vi "Gen - Poup Key in Sequence.vi"(6 "Type":enum16{"Error", "Info"}(ring)=enum."Info", 8 "Error in":errorcluster, 9 "Button text":string[](array[string])=["YES", "NO"], 10 "Data in":string[](array[string])) -> (0 "Error out":errorcluster, 2 "Data Out":T1, 3 "Yes?":bool)   [LabVIEW 2020]
uses:
  Control/State - eFGV.ctl
panel:
  in  "Section":string
  in  "Max blowdown pressure (psi)":string
  in  "Actuator pressure (psi)":string
  in  "Blowdown (Y/N)":string
  in  "Chart scale":string
  in  "Holding Time":string
  in  "Cycle":string(combo)
  in  "Test Pressure (psi)":string
  in  "Test Bunker":string(combo)
  in  "Test Media":string
  in  "Test Procedure":string
  in  "Variance":string
  in  "Test Req.":string
  in  "Test Req. ID":string
  in  "Test Sequence":string
  in  "Current File name":string
  out "procedure no./ref.  filename":string
  in  "Template Name":string
  out "Type Error":bool
  in  "No":bool
  in  "Yes":bool
  in  "Cancel":bool
  out "Type Info":bool
  in  "OK":bool
  out "Header out":string
  in  "Exit":bool
  out "Message":string
  in  "Auto Close?":bool
  in  "Message in":string
  in  "Header":string
  # "Sequence Parameter"
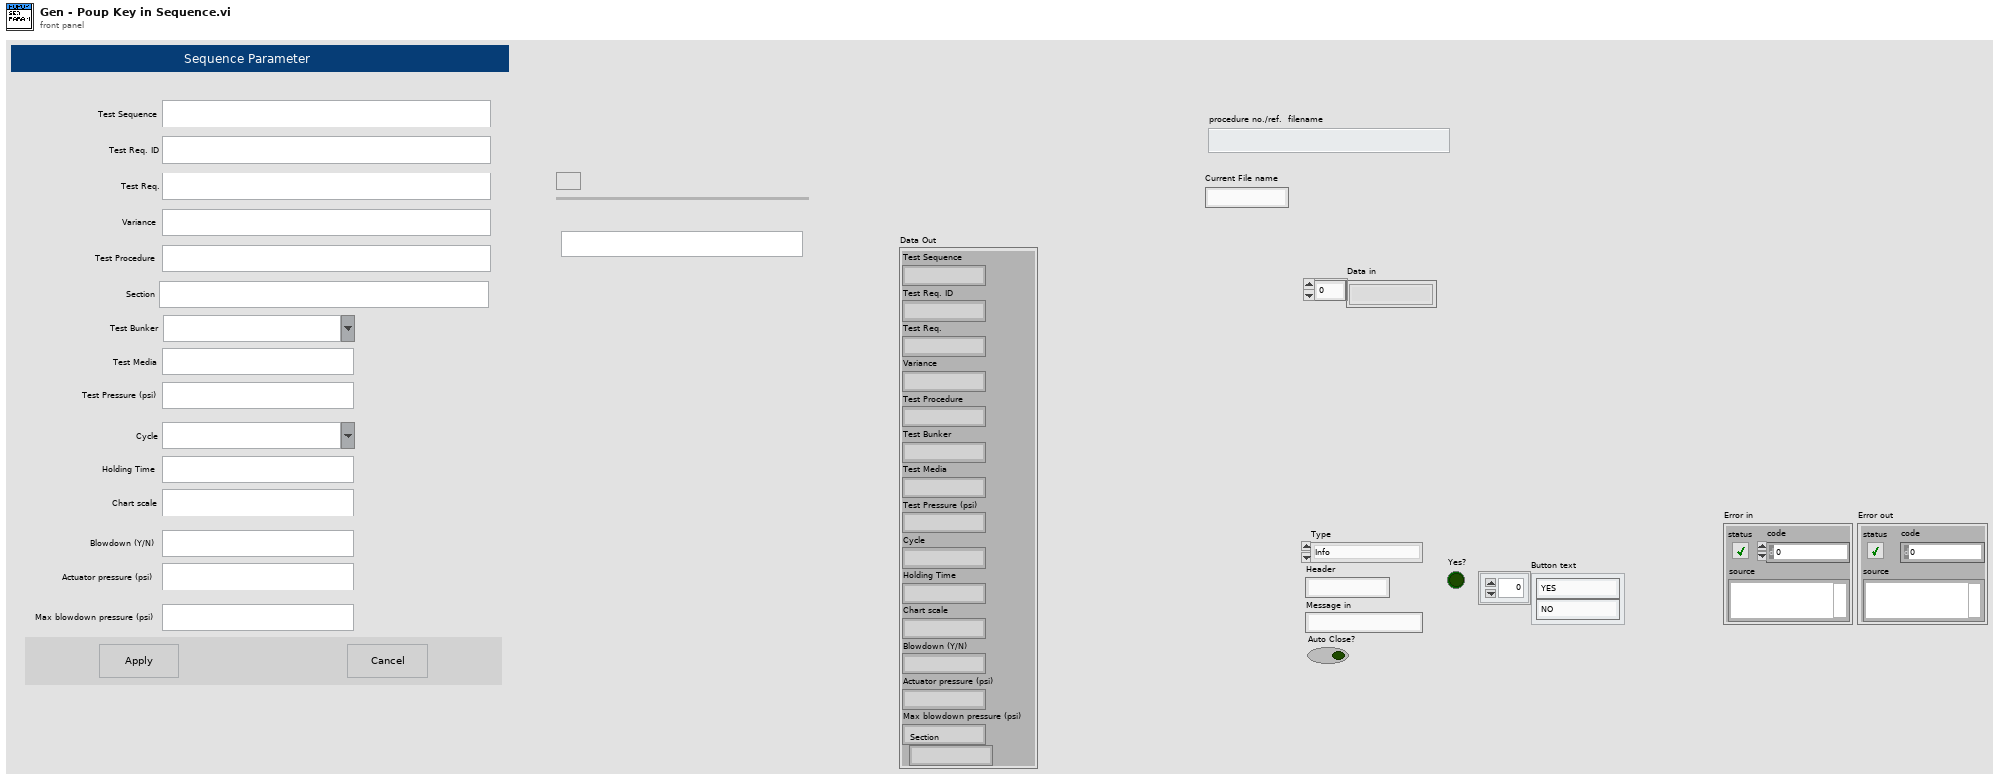
[diagram p1: front panel]
types:
  T1 = cluster{"Test Sequence":string, "Test Req. ID":string, "Test Req.":string, "Variance":string, "Test Procedure":string, "Test Bunker":string, "Test Media":string, "Test Pressure (psi)":string, "Cycle":string, "Holding Time":string, "Chart scale":string, "Blowdown (Y/N)":string, "Actuator pressure (psi)":string, "Max blowdown pressure (psi)":string, "Section":string}
  T2 = typedef "State - eFGV.ctl" = enum16{"Init", "Read", "Write", "Exit"}
  T3 = enum32{"Invalid", "Default", "Floating", "Floating/Auto-Hide", "Modal"}
  T4 = enum8{"Enabled", "Disabled", "Disabled and Grayed Out"}
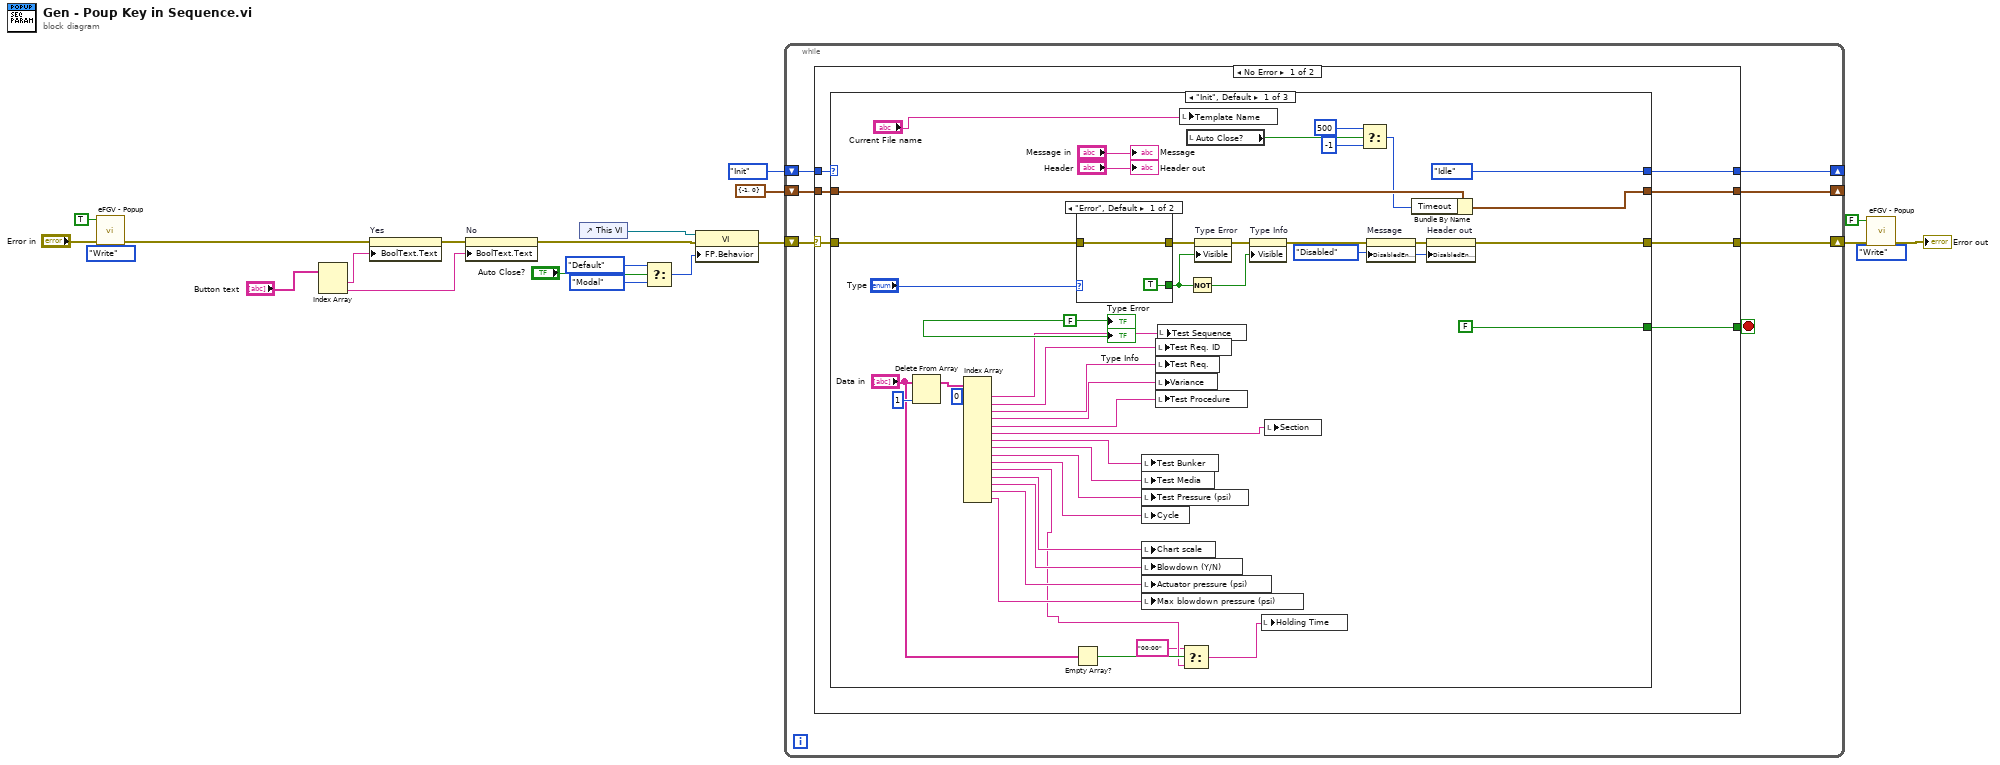
[diagram p0: block diagram]
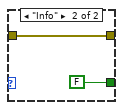
[diagram p2: hidden frame]
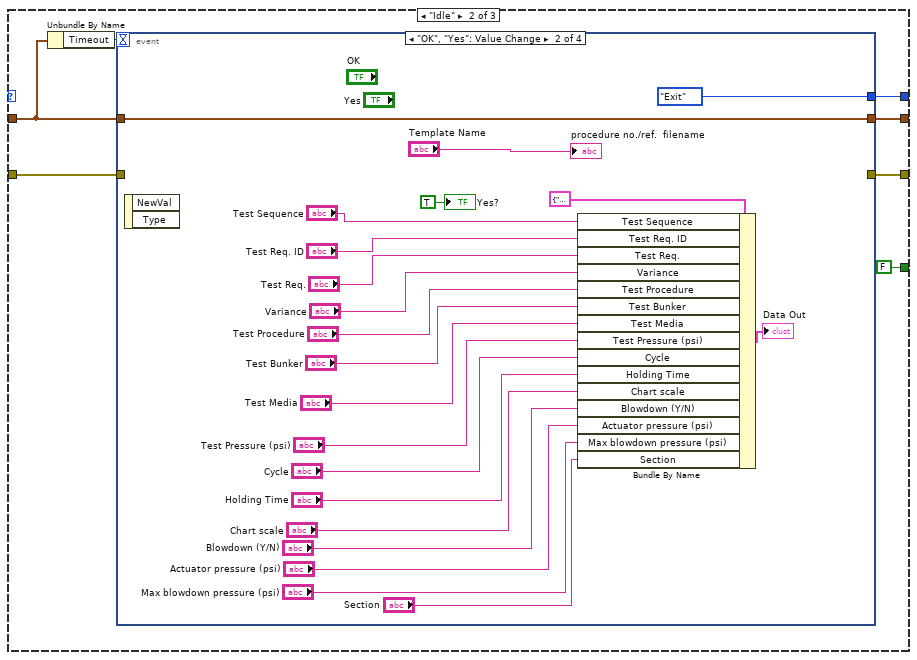
[diagram p3: hidden frame]
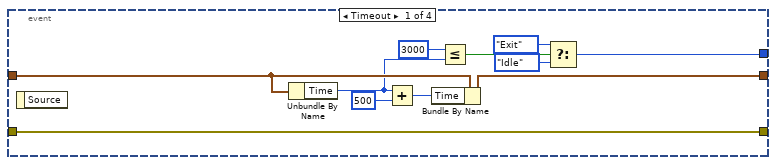
[diagram p4: hidden frame]
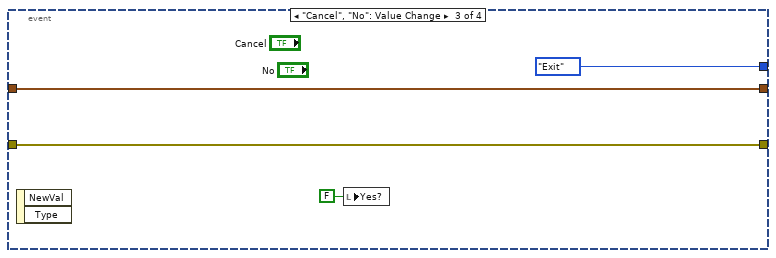
[diagram p5: hidden frame]
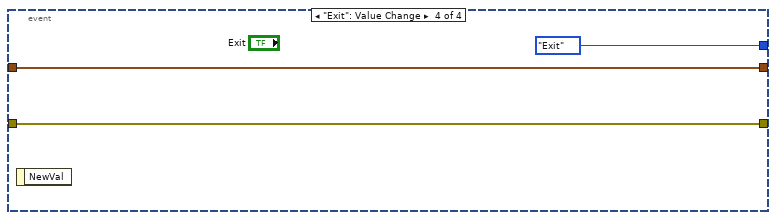
[diagram p6: hidden frame]
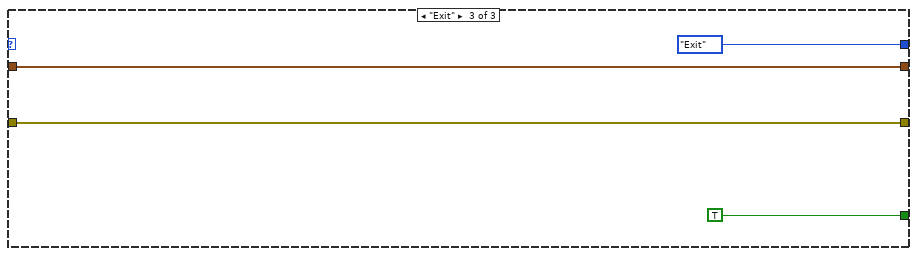
[diagram p7: hidden frame]
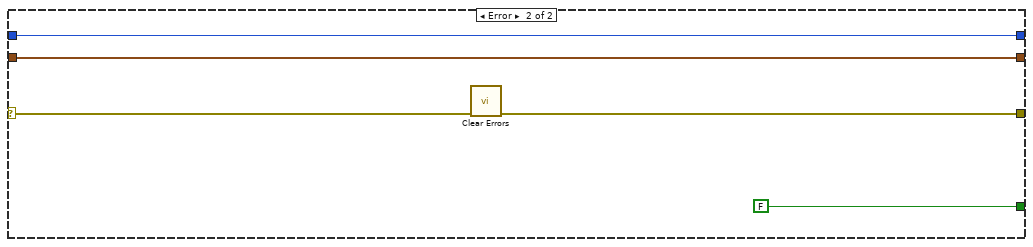
[diagram p8: hidden frame]
diagram:
  n1 = call "eFGV - Popup.vi"("Action"=State_-_eFGV."Write", "Error In"="Error in", "Popup"=TRUE) -> ("Error Out"=w1:errorcluster)  [unwired: 6 in, 2 out]
  n2 = Index Array(array="Button text") -> (element #1=w10:string, element #2=w9:string)  [unwired: 2 in]
  n3 = property on="Yes" class="Bool"(error in=w1, "BoolText.Text"=w10) -> (error out=w13:errorcluster)  [unwired: 1 in, 1 out]
  n4 = property on="No" class="Bool"(error in=w13, "BoolText.Text"=w9) -> (error out=w12:errorcluster)  [unwired: 1 in, 1 out]
  n5 = control-ref of="This VI"() -> (w19:refnum<vi>)
  n6 = Select(t=T3."Default" ("Front Panel Window:Behavior"), s="Auto Close?", f=T3."Modal") -> (s? t:f=w15:T3)
  n7 = property class="VI"(reference=w19, error in=w12, "FP.Behavior"=w15) -> (error out=w18:errorcluster)  [unwired: 1 out]
  n8 = while {
    shift-right: [w26] -> _
    shift-left: enum16{"Init", "Idle", "Exit"}."Init" -> [w27]
    shift-right: [w25] -> w5
    shift-left: w18 -> [w28]
    shift-right: [w22] -> _
    shift-left: cluster{"Timeout":i32, "Time":i32} {"Timeout"=-1, "Time"=0} -> [w23]
    stop <- w24 stop-if-true
    n9 = case shown="No Error" w28 {
      selector: w28 -> [w32 w137]
      tunnel: w27 -> [w35 w138]
      tunnel: [w34 w138] -> w26
      tunnel: [w33 w135] -> w25
      tunnel: [w31 FALSE] -> w24
      tunnel: w23 -> [w30 w134]
      tunnel: [w29 w134] -> w22
      frame No Error {
        n10 = case shown="\"Init\", Default" w35 {
          tunnel: [enum16{"Init", "Idle", "Exit"}."Idle" w90 enum16{"Init", "Idle", "Exit"}."Exit"] -> w34
          tunnel: [w64 w89 w133] -> w33
          tunnel: w32 -> [w71 w88 w133]
          tunnel: [FALSE FALSE TRUE] -> w31
          tunnel: w30 -> [w75 w85 w130]
          tunnel: [w74 w86 w130] -> w29
          frame "Init", Default {
            w67 = T4."Disabled" ("Disabled")
            w59 = FALSE ("Type Error")
            n11 = Delete From Array(array="Data in", index=1) -> (array with subset deleted=w56:string[])  [unwired: 1 in, 1 out]
            n12 = Index Array(array=w56, index #1=0 ("index")) -> (element #1=w54:string, element #2=w53:string, element #3=w52:string, element #4=w51:string, element #5=w50:string, element #6=w49:string, element #7=w48:string, element #8=w47:string, element #9=w46:string, element #10=w45:string, element #11=w37:string, element #12=w44:string, element #13=w43:string, element #14=w42:string, element #15=w41:string)  [unwired: 14 in]
            n13 = Empty Array?(array="Data in") -> (empty?=w39:bool)
            n14 = case shown="\"Error\", Default" "Type" {
              tunnel: [w80 w83] -> w72
              tunnel: w71 -> [w80 w83]
              tunnel: [TRUE FALSE] -> w69
              frame "Error", Default {
              }
              frame "Info" {
              }
            }
            n15 = local write "Test Bunker"(w48) -> ()
            n16 = local write "Test Media"(w47) -> ()
            n17 = local write "Test Pressure (psi)"(w46) -> ()
            n18 = local write "Cycle"(w45) -> ()
            n19 = local write "Chart scale"(w44) -> ()
            n20 = local write "Blowdown (Y/N)"(w43) -> ()
            n21 = local write "Actuator pressure (psi)"(w42) -> ()
            n22 = local write "Max blowdown pressure (psi)"(w41) -> ()
            n23 = local write "Test Req. ID"(w53) -> ()
            n24 = local write "Test Req."(w52) -> ()
            n25 = local write "Variance"(w51) -> ()
            n26 = local write "Test Procedure"(w50) -> ()
            n27 = local write "Test Sequence"(w54) -> ()
            n28 = local write "Template Name"("Current File name") -> ()
            n29 = Select(t="00:00", s=w39, f=w37) -> (s? t:f=w38:string)
            n30 = local read "Auto Close?"() -> (w60:bool)
            n31 = Not(x=w69) -> (.not. x?=w68:bool)
            n32 = property on="Type Error" class="Bool"(error in=w72, "Visible"=w69) -> (error out=w73:errorcluster)  [unwired: 1 in, 1 out]
            n33 = property on="Type Info" class="Bool (strict)"(error in=w73, "Visible"=w68) -> (error out=w65:errorcluster)  [unwired: 1 in, 1 out]
            n34 = local write "Holding Time"(w38) -> ()
            n35 = local write "Section"(w49) -> ()
            n36 = Select(t=500 ("Timeout"), s=w60, f=-1 ("Timeout")) -> (s? t:f=w62:i32)
            n37 = property on="Message" class="Str"(error in=w65, "DisabledEnum"=w67) -> (error out=w66:errorcluster)  [unwired: 1 in, 1 out]
            n38 = Bundle By Name(cluster=w75, "Timeout"=w62) -> (w74:cluster{"Timeout":i32, "Time":i32})
            n39 = property on="Header out" class="Str"(error in=w66, "DisabledEnum"=w67) -> (error out=w64:errorcluster)  [unwired: 1 in, 1 out]
            "Message" <- "Message in"
            "Header out" <- "Header"
            "Type Info" <- w59
            "Type Error" <- w59
          }
          frame "Idle" {
            n40 = Unbundle By Name(w85) -> ("Timeout"=w84:i32)
            n41 = event shown="[1] \"OK\", \"Yes\": Value Change" {
              selector: _ -> [_ _ _ _]
              dyn-events: _ -> [_ _ _ _]
              timeout: w84 -> [_ _ _ _]
              tunnel: [w93 enum16{"Init", "Idle", "Exit"}."Exit" enum16{"Init", "Idle", "Exit"}."Exit" enum16{"Init", "Idle", "Exit"}."Exit"] -> w90
              tunnel: [w101 _ w124 w127] -> w89
              tunnel: w88 -> [w101 _ w124 w127]
              tunnel: [w99 w122 w125 w128] -> w86
              tunnel: w85 -> [w100 w122 w125 w128]
              event Timeout {
                n42 = event-data() -> ()  [unwired: 1 in, 1 out]
                n43 = Unbundle By Name(w100) -> ("Time"=w96:i32)
                n44 = Add(x=w96, y=500) -> (x+y=w98:i32)
                n45 = Bundle By Name(cluster=w100, "Time"=w98) -> (w99:cluster{"Timeout":i32, "Time":i32})
                n46 = Less Or Equal?(x=3000, y=w96) -> (x <= y?=w94:bool)
                n47 = Select(t=enum16{"Init", "Idle", "Exit"}."Exit", s=w94, f=enum16{"Init", "Idle", "Exit"}."Idle") -> (s? t:f=w93:enum16{"Init", "Idle", "Exit"})
              }
              event "OK", "Yes": Value Change {
                n48 = event-data() -> ()  [unwired: 1 in, 2 out]
                n49 = Bundle By Name(cluster=T1 {"Test Sequence"="", "Test Req. ID"="", "Test Req."="", "Variance"="", "Test Procedure"="", "Test Bunker"="", "Test Media"="", "Test Pressure (psi)"="", "Cycle"="", "Holding Time"="", "Chart scale"="", "Blowdown (Y/N)"="", "Actuator pressure (psi)"="", "Max blowdown pressure (psi)"="", "Section"=""}, "Test Sequence"="Test Sequence", "Test Req. ID"="Test Req. ID", "Test Req."="Test Req.", "Variance"="Variance", "Test Procedure"="Test Procedure", "Test Bunker"="Test Bunker", "Test Media"="Test Media", "Test Pressure (psi)"="Test Pressure (psi)", "Cycle"="Cycle", "Holding Time"="Holding Time", "Chart scale"="Chart scale", "Blowdown (Y/N)"="Blowdown (Y/N)", "Actuator pressure (psi)"="Actuator pressure (psi)", "Max blowdown pressure (psi)"="Max blowdown pressure (psi)", "Section"="Section") -> (→"Data Out":T1)
                "Yes?" <- TRUE ("Yes?")
                "procedure no./ref.  filename" <- "Template Name"
              }
              event "Cancel", "No": Value Change {
                n50 = event-data() -> ()  [unwired: 1 in, 2 out]
                n51 = local write "Yes?"(FALSE ("Yes?")) -> ()
              }
              event "Exit": Value Change {
                n52 = event-data() -> ()  [unwired: 1 in, 1 out]
              }
            }
          }
          frame "Exit" {
          }
        }
      }
      frame Error {
        n53 = call <vilib>:"Clear Errors.vi"("error in (no error)"=w137) -> ("error out"=w135:errorcluster)  [unwired: 5 in, 1 out]
      }
    }
  }
  n54 = call "eFGV - Popup.vi"("Action"=State_-_eFGV."Write", "Error In"=w5, "Popup"=FALSE) -> ("Error Out"=→"Error out":errorcluster)  [unwired: 6 in, 2 out]
